vi "Event Driver.vi"(0 "event data":i32, 11 "error out":errorcluster, 13 "Operations":T1) -> (4 "Stop":refnum<user-event>, 15 "error out 2":errorcluster)   [LabVIEW 2020]
doc: "This VI handles User Events. It acts as a User Event Driver."
uses:
  Typedefs/Event Operations.ctl
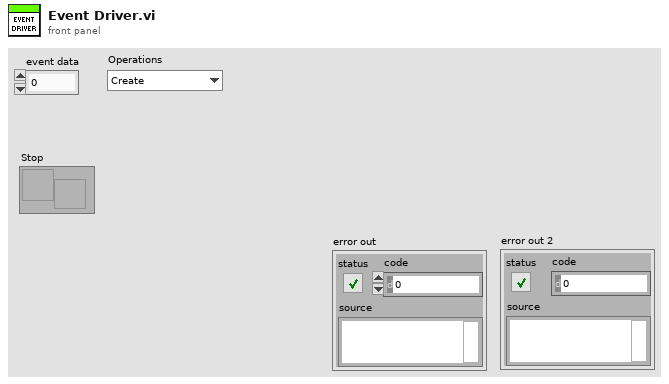
[diagram p1: front panel]
types:
  T1 = typedef "Event Operations.ctl" = enum16{"Create", "Generate", "Destroy"}
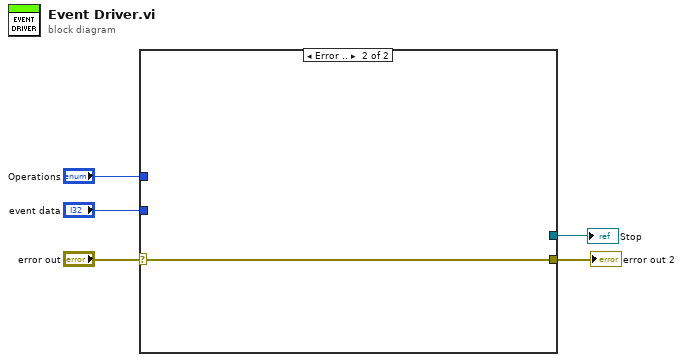
[diagram p0: block diagram]
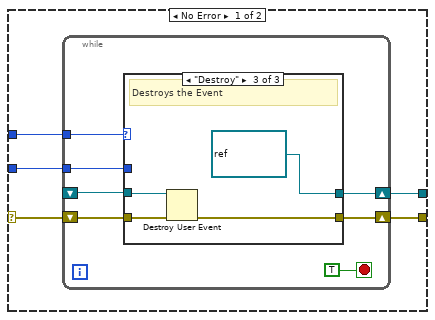
[diagram p2: hidden frame]
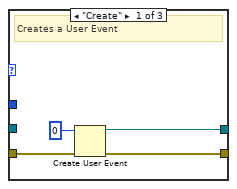
[diagram p3: hidden frame]
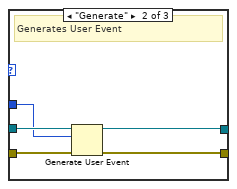
[diagram p4: hidden frame]
diagram:
  n1 = case shown="Error .." "error out" {
    selector: "error out" -> [w9 w31]
    tunnel: "Operations" -> [w10 _]
    tunnel: [w8 w31] -> w3
    tunnel: [w7 _] -> w2
    tunnel: "event data" -> [w6 _]
    frame No Error {
      n2 = while {
        tunnel: w10 -> [w17]
        shift-right: [w14] -> w8
        shift-left: w9 -> [w16]
        shift-right: [w13] -> w7
        shift-left: _ -> [w12]
        tunnel: w6 -> [w11]
        stop <- TRUE stop-if-true
        n3 = case shown="\"Destroy\"" w17 {
          tunnel: w16 -> [w21 w26 w30]
          tunnel: [w20 w25 w29] -> w14
          tunnel: [w18 w23 refnum<user-event> refnum ("user event")] -> w13
          tunnel: w12 -> [_ w24 w27]
          tunnel: w11 -> [_ w22 _]
          frame "Create" {
            # "Creates a User Event"
            n4 = Create User Event(user event datatype=0 ("Numeric"), error in=w21) -> (user event=w18:refnum<user-event>, error out=w20:errorcluster)
          }
          frame "Generate" {
            # "Generates User Event"
            n5 = Generate User Event(user event=w24, event data cluster=w22, error in=w26) -> (user event out=w23:refnum<user-event>, error out=w25:errorcluster)  [unwired: 1 in]
          }
          frame "Destroy" {
            # "Destroys the Event"
            n6 = Destroy User Event(user event=w27, error in=w30) -> (error out=w29:errorcluster)
          }
        }
      }
    }
    frame Error {
    }
  }
  "error out 2" <- w3
  "Stop" <- w2
